vi "Low rep rate beam pointing correction from kHz images_TBDEL.vi"() -> ()   [LabVIEW 2020]
doc: "The Parallel Processing (Optimized Performance) example shows how to process multiple images in parallel when using a ring acquisition. Images acquired from a camera are stored in a ring buffer and references to each image are pushed to a queue. Each worker loop removes a reference from the queue and processes the image.\n\nIn this example, image processing is simulated by a time delay that can be adjusted while the VI is running. When processing is complete, <B>IMAQdx Release Image</B> must be called in order to free space in the ring buffer."
uses:
  <vilib>/vision/Image Controls.llb/IMAQ Image.ctl
  tdms options.ctl
  C:/GEECS/Developers Version/source/Device Drivers/Point Grey Camera/fast camera acquisition/Thorlabs.MotionControl.Controls.dll
  Thorlabs.MotionControl.Controls.dll
  <vilib>/vision/driver/IMAQdx.llb/IMAQdx Acquisition Mode.ctl
  <vilib>/vision/driver/IMAQdx.llb/IMAQdx Buffer Number Mode.ctl
  C:/GEECS/Developers Version/source/Device Drivers/Point Grey Camera/fast camera acquisition/Thorlabs.MotionControl.KCube.PiezoCLI.dll
  Thorlabs.MotionControl.KCube.PiezoCLI.dll
  <vilib>/numeric/Random Number (Range) DBL.vi
  <vilib>/vision/driver/NI_Vision_Acquisition_Software.lvlib
  <resource>/objmgr/imaqdx.rc
panel:
  in  "SerialNumber":string
  in  "KCubePiezoControl":refnum<k24>(container)
  in  "Tab Control":enum32{"Main", "Instructions", "Errors"}(tab)
  in  "Camera Name":refnum<k21> caption="IMAQdx Session"
  out "Images in Queue":i32
  in  "# Images in Burst":i32=520
  out "Lost Buffer Count":u32
  out "Images Behind":u32
  out "Loop time":i32
  in  "Python version":string="3.6"
  in  "Enable Python":bool
  in  "Python module path":path
  out "Image":T1(plugin-control)
  in  "Stop":bool
  in  "Save":T2
  in  "min loop time per burst":u32=800
  out "error out":errorcluster
  out "acq error":errorcluster
  out "Python error":errorcluster
  out "unused buffers":T3(array[cluster])
  # "Requirements: Vision Acquisition Software\nInstructions:\nSet up the camera in NI max (exposure time, trigger mode, 8 bit, etc)\nSet all controls before running program\nSelect the Camera Name\nSelect # Images in burst\nRun the VI\n\n\nNotes:\nRecommended image size for 1kHz is 192x192 pix"
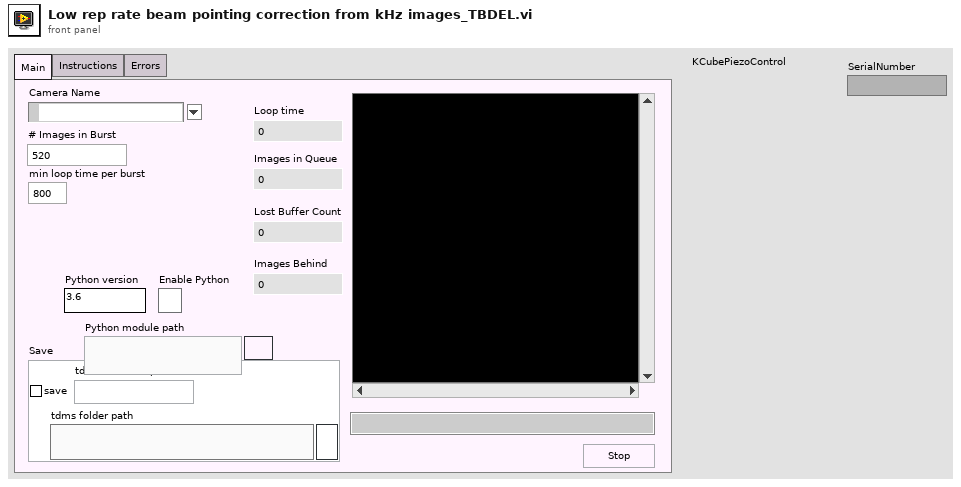
[diagram p1: front panel]
types:
  T1 = typedef "IMAQ Image.ctl" = refnum<image>
  T2 = typedef "tdms options.ctl" = cluster{"save":bool, "tdms filename prefix":string, "tdms folder path":path}
  T3 = cluster{"Image Out":T1, "Buffer Number Out":u32}[]
  T4 = typedef "IMAQdx.ctl" = refnum<k21>
  T5 = typedef "NI_Vision_Acquisition_Software.lvlib/IMAQdx Acquisition Mode.ctl" = enum32{"One Shot", "Continuous"}
  T6 = typedef "NI_Vision_Acquisition_Software.lvlib/IMAQdx Buffer Number Mode.ctl" = enum32{"Next", "Last", "Buffer Number", "Every", "Last New"}
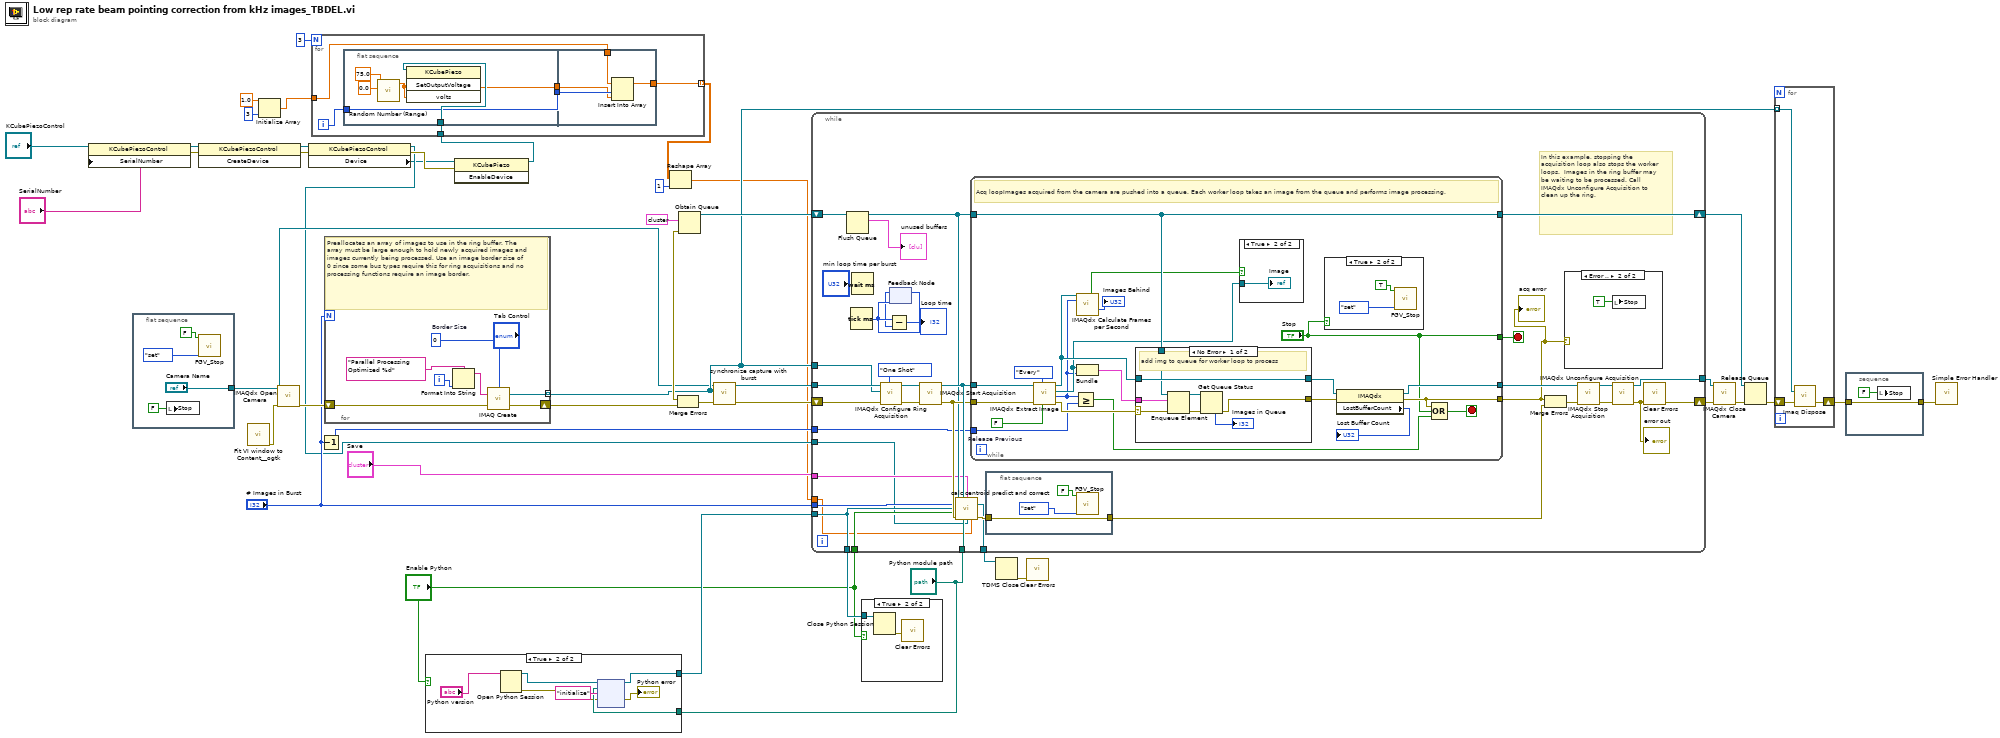
[diagram p0: block diagram]
diagram:
  n1 = property class="KCubePiezoControl"(reference="KCubePiezoControl", "SerialNumber"="SerialNumber") -> (reference out=w16:refnum<k24>, error out=w15:errorcluster)  [unwired: 1 in]
  n2 = flat-sequence {
    tunnel: ["Camera Name"] -> w43
    frame #0 {
      n3 = local write "Stop"(FALSE ("Stop")) -> ()
      n4 = call "FGV_Stop.vi"("command"=enum16{"set", "get"}."set", "stop"=FALSE) -> ()  [unwired: 9 in, 1 out]
    }
  }
  n5 = invoke class="KCubePiezoControl" method="CreateDevice"(reference=w16, error in=w15) -> (reference out=w12:refnum<k24>, error out=w14:errorcluster)  [unwired: 1 in, 1 out]
  n6 = call <userlib>:"Fit VI window to Content__ogtk.vi"() -> ("error out"=w23:errorcluster)  [unwired: 6 in, 1 out]
  n7 = Initialize Array(1.0 ("element"), 3 ("dimension size")) -> (w8:dbl[])
  n8 = call <vilib>:"IMAQdx Open Camera.vi"("error in"=w23, "Session In"=w43) -> ("error out"=w42:errorcluster, "Session Out"=w29:T4)  [unwired: 1 in, 7 out]
  n9 = property class="KCubePiezoControl"(reference=w12, error in=w14) -> (reference out=w7:refnum<k24>, error out=w13:errorcluster, "Device"=w6:refnum<k24>)
  n10 = Decrement(x="# Images in Burst") -> (x-1=w32:i32)
  n11 = for {
    N: "# Images in Burst" -> [_]
    tunnel: [w55] -> w30 mode=indexing
    shift-right: [w54] -> w40
    shift-left: w42 -> [w56]
    i -> [w53]
    w50 = 0  # Border Size
    # "Preallocates an array of images to use in the ring buffer. The array must be large enough to hold newly acquired images and images currently being processed. Use an image border size of 0 since some bus types require this for ring acquisitions and no processing functions require an image border."
    n12 = Format Into String(format string="Parallel Processing Optimized %d" ("Image Name"), w53) -> (resulting string=w52:string)  [unwired: 2 in, 1 out]
    n13 = call "IMAQ Create"("Border Size"=w50, "Image Name"=w52, "error in (no error)"=w56) -> ("New Image"=w55:T1, "error out"=w54:errorcluster)  [unwired: 1 in, 1 out]
  }
  n14 = case shown="True" "Enable Python" {
    tunnel: [_ w61] -> w25
    tunnel: "Python module path" -> [_ w59]
    frame False {
    }
    frame True {
      n15 = Open Python Session(python version="Python version") -> (session out=w62:refnum<k35>, error out=w58:errorcluster)  [unwired: 2 in]
      n16 = node(w62, w59, "initialize" ("function name"), w58) -> (w61:refnum<k35>, →"Python error":errorcluster)  [unwired: 2 in, 2 out]
    }
  }
  n17 = invoke class="KCubePiezo" method="EnableDevice"(reference=w6, error in=w13) -> (reference out=w5:refnum<k24>)  [unwired: 1 in, 2 out]
  n18 = for {
    N: 3 -> [_]
    tunnel: w8 -> [w65]
    tunnel: w5 -> [w69]
    tunnel: [w64] -> w3 mode=indexing
    i -> [w68]
    n19 = flat-sequence {
      tunnel: w69 -> [w72]
      tunnel: w68 -> [w71]
      tunnel: [w71] -> w67
      tunnel: [w70] -> w66
      tunnel: w67 -> [w78]
      tunnel: w66 -> [w77]
      tunnel: w65 -> [w76]
      tunnel: [w75] -> w64
      frame #0 {
        n20 = call-poly <vilib>:"Random Number (Range).vi"("lower bound (0)"=0.0, "upper bound (100)"=75.0) -> ("number"=w70:dbl)  [unwired: 9 in]
        n21 = invoke class="KCubePiezo" method="SetOutputVoltage"(reference=w72, "volts"=w70) -> ()  [unwired: 2 in, 4 out]
      }
      frame #1 {
        n22 = Insert Into Array(array=w76, index=w78, new element=w77) -> (w75:dbl[])
      }
    }
  }
  n23 = Reshape Array(w3, 1 ("dimension size")) -> (w1:dbl[])
  n24 = Obtain Queue(element data type=cluster{"Image Out":T1, "Buffer Number Out":u32} {"Image Out"=refnum, "Buffer Number Out"=0}) -> (queue out=w36:refnum<queue>, error out=w39:errorcluster)  [unwired: 4 in, 1 out]
  n25 = Merge Errors(w39, w40) -> (w26:errorcluster)
  n26 = call "synchronize capture with burst.vi"("error in (no error)"=w26, "Image Array"=w30, "Refnum in"=w29) -> ("error out"=w28:errorcluster, "Refnum out"=w27:T4)  [unwired: 7 in]
  n27 = while {
    tunnel: w27 -> [w114]
    tunnel: w30 -> [w111]
    shift-right: [w89] -> w33
    shift-left: w28 -> [w113]
    shift-right: [w112] -> w38
    shift-left: w36 -> [w110]
    tunnel: [w90] -> w35
    tunnel: w32 -> [w88]
    tunnel: "# Images in Burst" -> [w87]
    tunnel: w25 -> [w86]
    tunnel: [w86] -> w24
    tunnel: "Enable Python" -> [w85]
    tunnel: "Python module path" -> [w84]
    tunnel: "Save" -> [w82]
    tunnel: [w81] -> w20
    tunnel: w7 -> [w80]
    tunnel: w1 -> [w79]
    stop <- w91 stop-if-true
    # "In this example, stopping the acquisition loop also stops the worker loops.  Images in the ring buffer may be waiting to be processed. Call IMAQdx Unconfigure Acquisition to clean up the ring."
    n28 = Flush Queue(queue=w110) -> (queue out=w93:refnum<queue>, remaining elements=→"unused buffers":T3)  [unwired: 1 in, 1 out]
    n29 = Tick Count (ms)() -> (millisecond timer value=w98:u32)
    n30 = Wait (ms)(milliseconds to wait="min loop time per burst") -> ()  [unwired: 1 out]
    n31 = call <vilib>:"IMAQdx Configure Ring Acquisition.vi"("Mode"=IMAQdx_Acquisition_Mode."One Shot" ("Continuous?"), "error in"=w113, "Images"=w111, "Session In"=w114) -> ("error out"=w106:errorcluster, "Session Out"=w107:T4)  [unwired: 5 in, 1 out]
    n32 = feedback #1(w98) -> (w97:u32)
    n33 = Subtract(x=w98, y=w97) -> (x-y=→"Loop time":u32)
    n34 = feedback-in #1(w98) -> ()
    n35 = call <vilib>:"IMAQdx Start Acquisition.vi"("error in"=w106, "Session In"=w107) -> ("error out"=w101:errorcluster, "Session Out"=w102:T4)  [unwired: 8 out]
    n36 = call "calc centroid predict and correct.vi"("Queue in"=w93, "Session Out"=w102, "Save"=w82, "# Images in Burst"=w87, "Python session"=w86, "Enable Python"=w85, "error in (no error)"=w101, "module path"=w84, "reference"=w80, "PIezo Voltages"=w79) -> ("tdms ref out"=w81:refnum<k34>, "error out"=w100:errorcluster)  [unwired: 3 in, 1 out]
    n37 = while {
      tunnel: w101 -> [w139]
      tunnel: w102 -> [w136]
      tunnel: w93 -> [w129]
      tunnel: [w135] -> w103
      tunnel: [w133] -> w83
      tunnel: [w129] -> w112
      tunnel: ["Stop"] -> w91
      tunnel: w88 -> [w121]
      stop <- w122 stop-if-true
      w137 = FALSE  # Release Previous
      # "Acq loopImages acquired from the camera are pushed into a queue. Each worker loop takes an image from the queue and performs image processing."
      n38 = call <vilib>:"IMAQdx Extract Image.vi"("Release Previous (true)"=w137, "Buffer Number Mode (Next)"=IMAQdx_Buffer_Number_Mode."Every" ("Buffer Number Mode"), "error in"=w139, "Session In"=w136) -> ("error out"=w132:errorcluster, "Buffer Number Out"=w123:u32, "Image Out"=w124:T1, "Session Out"=w126:T4)  [unwired: 4 in]
      n39 = Greater Or Equal?(x=w123, y=w121) -> (x >= y?=w120:bool)
      n40 = call <vilib>:"IMAQdx Calculate Frames per Second.vi"("Session In"=w126, "Buffer Number"=w123) -> ("Update Display"=w125:bool, "Images Behind"=→"Images Behind":i32)  [unwired: 7 in, 5 out]
      n41 = Bundle("Image Out"=w124, "Buffer Number Out"=w123) -> (w130:cluster{"Image Out":T1, "Buffer Number Out":u32})  [unwired: 1 in]
      n42 = case shown="No Error" w132 {
        selector: w132 -> [w146 w151]
        tunnel: [w147 w152] -> w131
        tunnel: w126 -> [w147 w152]
        tunnel: w130 -> [w145 _]
        tunnel: w129 -> [w144 _]
        tunnel: [w143 w151] -> w128
        frame No Error {
          # "add img to queue for worker loop to process"
          n43 = Enqueue Element(queue=w144, element=w145, error in (no error)=w146) -> (queue out=w149:refnum<queue>, error out=w150:errorcluster)  [unwired: 1 in, 1 out]
          n44 = Get Queue Status(queue=w149, error in (no error)=w150) -> (error out=w143:errorcluster, # elements in queue=→"Images in Queue":i32)  [unwired: 1 in, 6 out]
        }
        frame Error {
        }
      }
      n45 = case shown="True" w125 {
        tunnel: w124 -> [_ w142]
        frame False {
        }
        frame True {
          "Image" <- w142
        }
      }
      n46 = case shown="True" "Stop" {
        frame False {
        }
        frame True {
          n47 = call "FGV_Stop.vi"("command"=enum16{"set", "get"}."set", "stop"=TRUE) -> ()  [unwired: 9 in, 1 out]
        }
      }
      n48 = property class="IMAQdx"(reference=w131, error in=w128) -> (reference out=w135:T4, error out=w133:errorcluster, "LostBufferCount"=→"Lost Buffer Count":u32)
      n49 = Compound Arithmetic op=OR(w133, "Stop", w120) -> (w122:bool)
    }
    "acq error" <- w83
    n50 = flat-sequence {
      tunnel: w100 -> [w116]
      tunnel: [w116] -> w99
      frame #0 {
        n51 = call "FGV_Stop.vi"("command"=enum16{"set", "get"}."set", "stop"=FALSE) -> ()  [unwired: 9 in, 1 out]
      }
    }
    n52 = Merge Errors(w83, w99) -> (w104:errorcluster)
    n53 = case shown="Error .." w83 {
      frame No Error {
      }
      frame Error {
        n54 = local write "Stop"(TRUE ("Stop")) -> ()
      }
    }
    n55 = call <vilib>:"IMAQdx Stop Acquisition.vi"("error in"=w104, "Session In"=w103) -> ("error out"=w108:errorcluster, "Session Out"=w109:T4)  [unwired: 8 out]
    n56 = call <vilib>:"IMAQdx Unconfigure Acquisition.vi"("error in"=w108, "Session In"=w109) -> ("error out"=w95:errorcluster, "Session Out"=w90:T4)  [unwired: 8 out]
    "error out" <- w95
    n57 = call <vilib>:"Clear Errors.vi"("error in (no error)"=w95) -> ("error out"=w89:errorcluster)  [unwired: 5 in, 1 out]
  }
  n58 = case shown="True" "Enable Python" {
    tunnel: w24 -> [_ w154]
    frame False {
    }
    frame True {
      n59 = Close Python Session(session in=w154) -> (11:w153:errorcluster)  [unwired: 1 in]
      n60 = call <vilib>:"Clear Errors.vi"("error in (no error)"=w153) -> ()  [unwired: 5 in, 2 out]
    }
  }
  n61 = TDMS Close(11:w20) -> (0:w21:errorcluster)  [unwired: 1 in, 1 out]
  n62 = call <vilib>:"Clear Errors.vi"("error in (no error)"=w21) -> ()  [unwired: 5 in, 2 out]
  n63 = call <vilib>:"IMAQdx Close Camera.vi"("error in"=w33, "Session In"=w35) -> ("error out"=w34:errorcluster)  [unwired: 9 out]
  n64 = Release Queue(queue=w38, error in (no error)=w34) -> (error out=w37:errorcluster)  [unwired: 1 in, 2 out]
  n65 = for {
    shift-right: [w156] -> w44
    shift-left: w37 -> [w157]
    tunnel: w30 -> [w155] mode=indexing
    n66 = call "Imaq Dispose"("Image"=w155, "error in (no error)"=w157) -> ("error out"=w156:errorcluster)  [unwired: 4 in]
  }
  n67 = stacked-sequence {
    tunnel: [w158] -> w45
    tunnel: w44 -> [w158]
    frame #0 {
      n68 = local write "Stop"(FALSE ("Stop")) -> ()
    }
  }
  n69 = call <vilib>:"Simple Error Handler.vi"("error in (no error)"=w45) -> ()  [unwired: 4 in, 5 out]
